vi "Config Zero Point.vi"(7 "Zero Single (off)":bool, 8 "error in":errorcluster, 9 "Loss Point (0 jpF)":dbl min=-99999999.0 max=99999999.0 format="%#_10f", 10 "Capacitance Point (0 pF)":dbl min=-99999999.0 max=99999999.0 format="%#_10f", 11 "VISA resource name":refnum<visa-resource-name>) -> (0 "error out":errorcluster, 3 "VISA resource name out":refnum<visa-resource-name>)   [LabVIEW 2016, in "Andeen-Hagerling 2550.lvlib"]
doc: "This vi provides manual and automatic ways to enter capacitance and loss Zero compensation values."
uses:
  Andeen-Hagerling 2550.lvlib
panel:
  # "Zero Point Parameters"
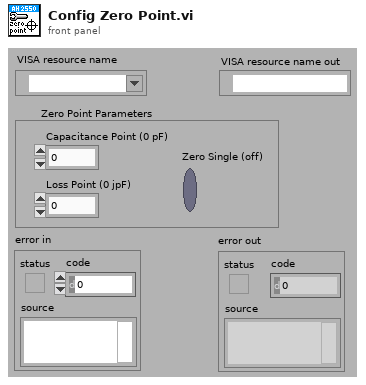
[diagram p1: front panel]
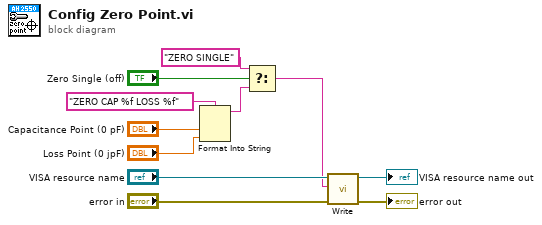
[diagram p0: block diagram]
diagram:
  n1 = Format Into String(format string="ZERO CAP %f LOSS %f", "Capacitance Point (0 pF)", "Loss Point (0 jpF)") -> (resulting string=w2:string)  [unwired: 2 in, 1 out]
  n2 = Select(t="ZERO SINGLE" ("format string"), s="Zero Single (off)", f=w2) -> (s? t:f=w1:string)
  n3 = call "Write.vi"("error in"="error in", "command"=w1, "VISA resource name"="VISA resource name") -> ("error out"=→"error out":errorcluster, "VISA resource name out"=→"VISA resource name out":refnum<visa-resource-name>)  [unwired: 7 in]
